vi "Vision2.vi"   [LabVIEW 2016]
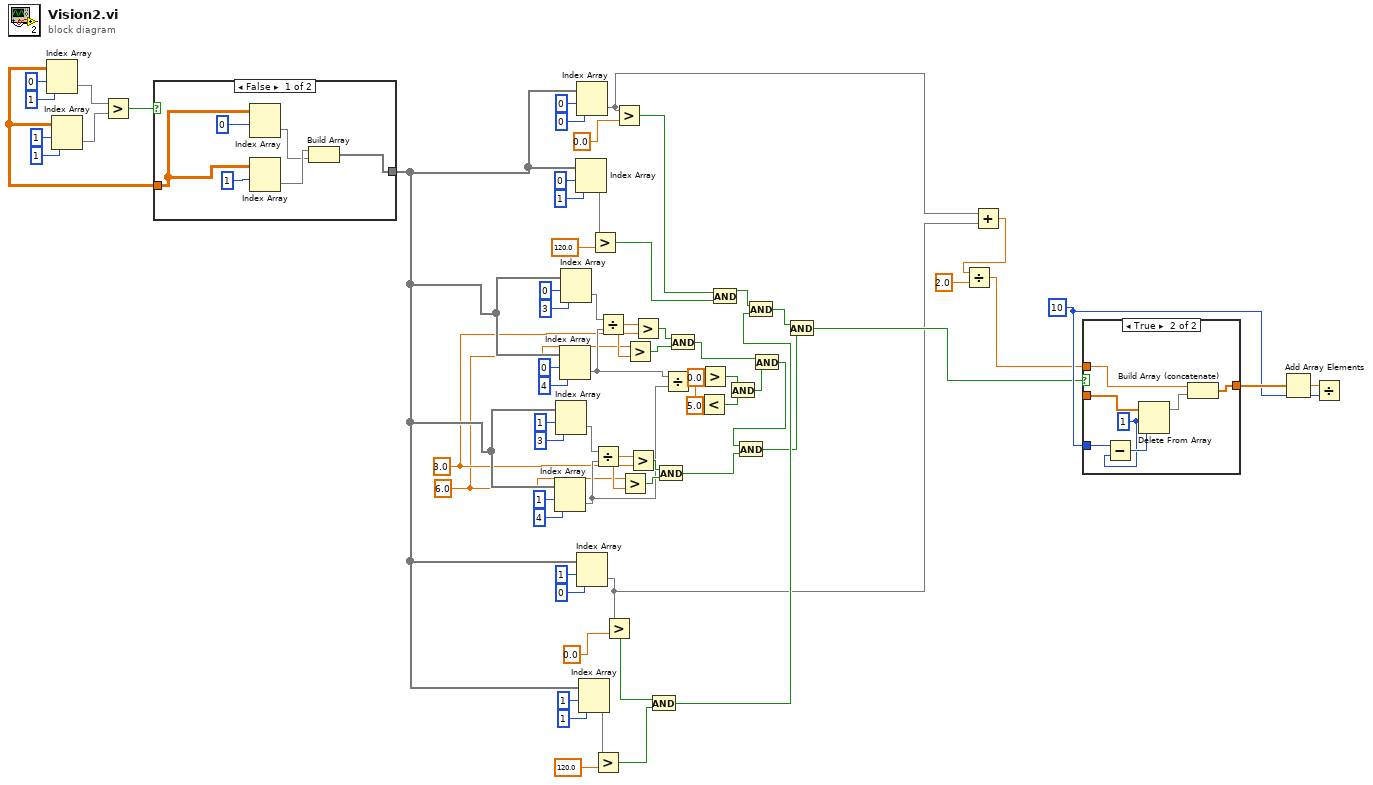
[diagram p0: block diagram]
diagram:
  w1 = 6.0 ("x")
  w2 = 3.0 ("y")
  w58 = 10
  n1 = Index Array(index (row)=0, index (col)=1 ("disabled index (col)")) -> (array=w4:dbl[][], element=w6)
  n2 = Index Array(array=w4, index (row)=1, index (col)=1 ("disabled index (col)")) -> (element=w7)
  n3 = Greater?(x=w6, y=w7) -> (0:w5:bool)
  n4 = case shown="False" w5 {
    tunnel: w4 -> [w76 w78]
    tunnel: [w72 w78] -> w3
    frame False {
      n5 = Index Array(array=w76, index (row)=0) -> (element=w73)  [unwired: 1 in]
      n6 = Index Array(array=w76, index (row)=1) -> (element=w74)  [unwired: 1 in]
      n7 = Build Array(w74, w73) -> (w72:void[])
    }
    frame True {
    }
  }
  n8 = Index Array(array=w3, index (row)=1, index (col)=4 ("disabled index (col)")) -> (element=w29)
  n9 = Index Array(array=w3, index (row)=1, index (col)=3 ("disabled index (col)")) -> (element=w34)
  n10 = Index Array(array=w3, index (row)=0, index (col)=4 ("disabled index (col)")) -> (element=w30)
  n11 = Index Array(array=w3, index (row)=0, index (col)=3 ("disabled index (col)")) -> (element=w42)
  n12 = Index Array(array=w3, index (row)=0, index (col)=1 ("disabled index (col)")) -> (element=w65)
  n13 = Index Array(array=w3, index (row)=0, index (col)=0 ("disabled index (col)")) -> (element=w13)
  n14 = Index Array(array=w3, index (row)=1, index (col)=0 ("disabled index (col)")) -> (element=w12)
  n15 = Index Array(array=w3, index (row)=1, index (col)=1 ("disabled index (col)")) -> (element=w52)
  n16 = Greater?(x=w65, y=120.0) -> (0:w62:bool)
  n17 = Divide(x=w34, y=w29) -> (x/y=w33:dbl)
  n18 = Greater?(x=w52, y=120.0) -> (0:w49:bool)
  n19 = Divide(x=w42, y=w30) -> (x/y=w41:dbl)
  n20 = Greater?(x=w12, y=0.0) -> (0:w50:bool)
  n21 = Greater?(x=w13, y=0.0) -> (0:w63:bool)
  n22 = Greater?(x=w1, y=w33) -> (0:w31:bool)
  n23 = Greater?(x=w1, y=w41) -> (0:w40:bool)
  n24 = Greater?(x=w33, y=w2) -> (0:w32:bool)
  n25 = Greater?(x=w41, y=w2) -> (0:w39:bool)
  n26 = And(x=w50, y=w49) -> (x .and. y?=w47:bool)
  n27 = And(x=w32, y=w31) -> (x .and. y?=w21:bool)
  n28 = Divide(x=w30, y=w29) -> (x/y=w26:dbl)
  n29 = And(x=w39, y=w40) -> (x .and. y?=w23:bool)
  n30 = Less?(x=w26, y=5.0) -> (x < y?=w24:bool)
  n31 = Greater?(x=w26, y=0.0) -> (0:w25:bool)
  n32 = And(x=w63, y=w62) -> (x .and. y?=w48:bool)
  n33 = And(x=w25, y=w24) -> (x .and. y?=w22:bool)
  n34 = And(x=w48, y=w47) -> (x .and. y?=w18:bool)
  n35 = And(x=w23, y=w22) -> (x .and. y?=w20:bool)
  n36 = And(x=w20, y=w21) -> (x .and. y?=w19:bool)
  n37 = And(x=w18, y=w19) -> (x .and. y?=w17:bool)
  n38 = Add(x=w13, y=w12) -> (x+y=w16:dbl)
  n39 = Divide(x=w16, y=2.0) -> (x/y=w15:dbl)
  n40 = case shown="True" w17 {
    tunnel: w15 -> [_ w86]
    tunnel: [w79 w85] -> w61
    tunnel: [w79 w83] -> w60
    tunnel: w58 -> [_ w80]
    frame False {
    }
    frame True {
      w81 = 1 ("length")
      n41 = Subtract(x=w80, y=w81) -> (x-y=w82:i32)
      n42 = Delete From Array(array=w83, length=w81, index=w82) -> (array with subset deleted=w84)  [unwired: 1 out]
      n43 = Build Array (concatenate)(w86, w84) -> (w85:dbl[])
    }
  }
  n44 = Add Array Elements(numeric array=w61) -> (sum=w69:dbl)
  n45 = Divide(x=w69, y=w58) -> (x/y=w59:dbl)
